vi "VNS IRH3T wOSSPClass.vi"(8 "error in (no error)":errorcluster, 10 "Best Chromosome In":u16[](array[numeric])=[1, 7, 8, 14, 6, 15, 11, 12, 3, 9, 5, 10, 4, 13, 0, 2], 11 "OSSP_Problem.lvclass":refnum<class "OSSP_Problem.lvclass">) -> (0 "error out":errorcluster, 1 "Tardiness(FIFO Engine)":u16, 2 "VNS Result":u16[](array[numeric]), 3 "OSSP_Problem out":refnum<class "OSSP_Problem.lvclass">)   [LabVIEW 2013]
uses:
  Classes/OSSP_Problem.lvclass
  Classes/OSSP_Problem.lvclass/OSSP_Problem.ctl
  GA/SubVIS/Remove Duplicates In Array.vi
  Classes/GanntChart_Class/Schedule and Create Gannt Chart.vi
  Classes/GanntChart_Class/Job Completion Times.vi
  Classes/GanntChart_Class/Reorder Chromosome  After Makespan Calculation.vi
  Classes/GanntChart_Class/Check Other Machines for Schedule Time.vi
  Classes/GanntChart_Class/Schedule Job.vi
  Classes/GanntChart_Class/Find Gaps on Particular Machine.vi
  Classes/GanntChart_Class/Increment Number of Jobs on Machine.vi
  Classes/GanntChart_Class/Operation to Machine Job Tuple.vi
  Classes/GanntChart_Class/Find Job On Other Machines.vi
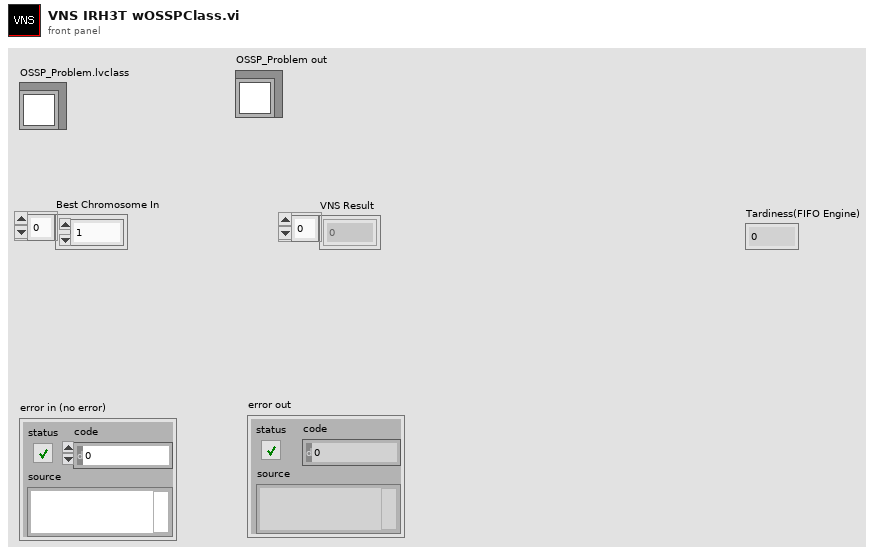
[diagram p1: front panel]
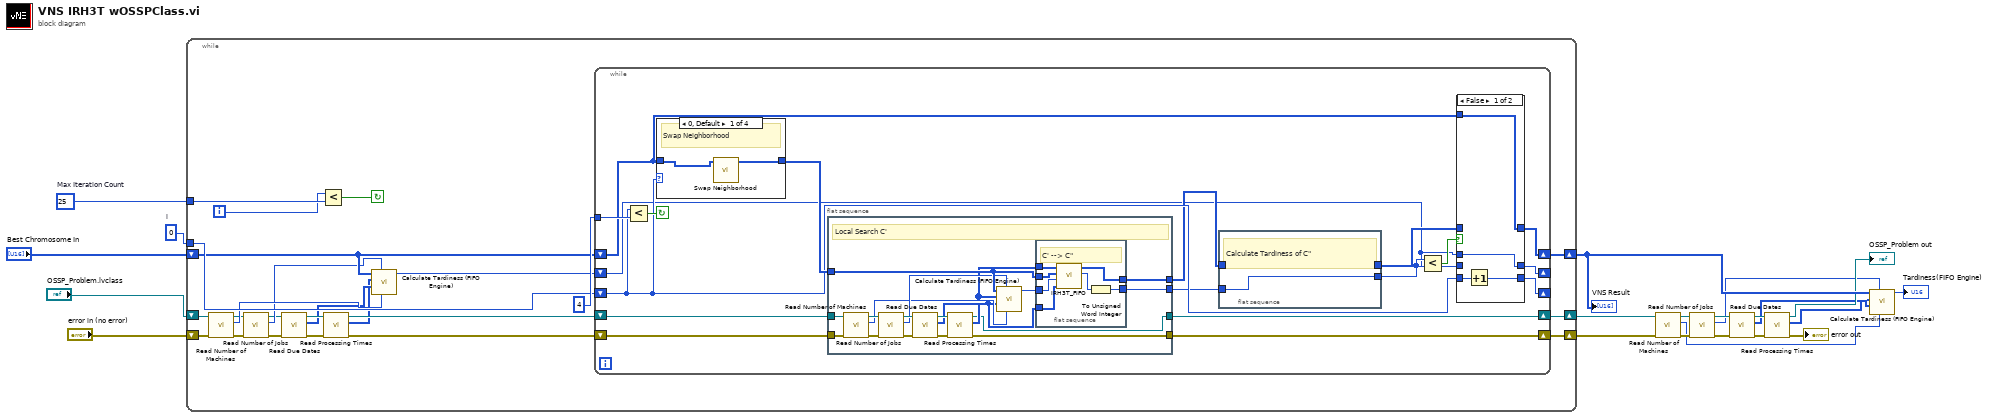
[diagram p0: block diagram]
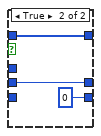
[diagram p2: hidden frame]
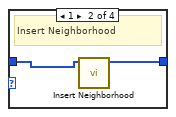
[diagram p3: hidden frame]
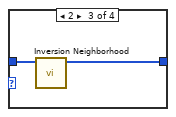
[diagram p4: hidden frame]
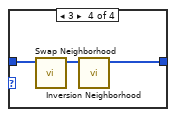
[diagram p5: hidden frame]
diagram:
  w20 = 0  # i
  w21 = 25  # Max Iteration Count
  n1 = while {
    tunnel: w21 -> [w45]
    tunnel: w20 -> [w42]
    shift-right: [w40] -> w19
    shift-left: "Best Chromosome In" -> [w33]
    shift-right: [w39] -> w10
    shift-left: "OSSP_Problem.lvclass" -> [w37]
    shift-right: [w38] -> w8
    shift-left: "error in (no error)" -> [w35]
    i -> [w41]
    stop <- w44 continue-if-true
    n2 = call-dynamic "Read Number of Machines.vi"("error in (no error)"=w35, "OSSP_Problem in"=w37) -> ("error out"=w30:errorcluster, "Number of Machines"=w32:i32, "OSSP_Problem out"=w31:refnum<class "OSSP_Problem.lvclass">)  [unwired: 7 in]
    n3 = call-dynamic "Read Number of Jobs.vi"("error in (no error)"=w30, "OSSP_Problem in"=w31) -> ("error out"=w27:errorcluster, "Number of Jobs"=w29:i32, "OSSP_Problem out"=w28:refnum<class "OSSP_Problem.lvclass">)  [unwired: 7 in]
    n4 = call "Read Due Dates.vi"("error in (no error)"=w27, "OSSP_Problem in"=w28) -> ("error out"=w26:errorcluster, "Due Dates"=w24:u16[], "OSSP_Problem out"=w25:refnum<class "OSSP_Problem.lvclass">)  [unwired: 7 in]
    n5 = Less?(x=w41, y=w45) -> (x < y?=w44:bool)
    n6 = call-dynamic "Read Processing Times.vi"("error in (no error)"=w26, "OSSP_Problem in"=w25) -> ("error out"=w34:errorcluster, "Processing Times"=w23:u16[][], "OSSP_Problem out"=w36:refnum<class "OSSP_Problem.lvclass">)  [unwired: 7 in]
    n7 = call "Calculate Tardiness (FIFO Engine).vi"("Number of Machines"=w32, "Number of Jobs"=w29, "Due Dates"=w24, "Processing Times"=w23, "Schedule In"=w33) -> ("Tardiness(FIFO Engine)"=w22:u16)  [unwired: 6 in]
    n8 = while {
      tunnel: 4 -> [w60]
      shift-right: [w59] -> _
      shift-left: w42 -> [w56]
      shift-right: [w58] -> w40
      shift-left: w33 -> [w57]
      shift-right: [w54] -> w39
      shift-left: w36 -> [w52]
      shift-right: [w53] -> w38
      shift-left: w34 -> [w51]
      shift-right: [w49] -> _
      shift-left: w22 -> [w46]
      stop <- w63 continue-if-true
      n9 = Less?(x=w56, y=w60) -> (x < y?=w63:bool)
      n10 = case shown="0, Default" w56 {
        tunnel: w57 -> [w99 w101 w103 w106]
        tunnel: [w98 w100 w102 w104] -> w62
        frame 0, Default {
          # "Swap Neighborhood"
          n11 = call "Swap Neighborhood.vi"("Schedule In"=w99) -> ("Schedule Out"=w98:u16[])  [unwired: 10 in]
        }
        frame 1 {
          # "Insert Neighborhood"
          n12 = call "Insert Neighborhood.vi"("C'"=w101) -> ("Best Chromosome In"=w100:u16[])  [unwired: 10 in]
        }
        frame 2 {
          n13 = call "Inversion Neighborhood.vi"("Schedule in"=w103) -> ("Schedule out"=w102:u16[])  [unwired: 10 in]
        }
        frame 3 {
          n14 = call "Swap Neighborhood.vi"("Schedule In"=w106) -> ("Schedule Out"=w105:u16[])  [unwired: 10 in]
          n15 = call "Inversion Neighborhood.vi"("Schedule in"=w105) -> ("Schedule out"=w104:u16[])  [unwired: 10 in]
        }
      }
      n16 = flat-sequence {
        tunnel: w62 -> [w89]
        tunnel: [w90] -> w48
        tunnel: [w87] -> w55
        tunnel: w52 -> [w80]
        tunnel: [w75] -> w54
        tunnel: w51 -> [w74]
        tunnel: [w73] -> w53
        frame #0 {
          # "Local Search C'"
          n17 = call-dynamic "Read Number of Machines.vi"("error in (no error)"=w74, "OSSP_Problem in"=w80) -> ("error out"=w85:errorcluster, "Number of Machines"=w78:i32, "OSSP_Problem out"=w86:refnum<class "OSSP_Problem.lvclass">)  [unwired: 7 in]
          n18 = call-dynamic "Read Number of Jobs.vi"("error in (no error)"=w85, "OSSP_Problem in"=w86) -> ("error out"=w83:errorcluster, "Number of Jobs"=w79:i32, "OSSP_Problem out"=w84:refnum<class "OSSP_Problem.lvclass">)  [unwired: 7 in]
          n19 = call "Read Due Dates.vi"("error in (no error)"=w83, "OSSP_Problem in"=w84) -> ("error out"=w82:errorcluster, "Due Dates"=w77:u16[], "OSSP_Problem out"=w81:refnum<class "OSSP_Problem.lvclass">)  [unwired: 7 in]
          n20 = call-dynamic "Read Processing Times.vi"("error in (no error)"=w82, "OSSP_Problem in"=w81) -> ("error out"=w73:errorcluster, "Processing Times"=w76:u16[][], "OSSP_Problem out"=w75:refnum<class "OSSP_Problem.lvclass">)  [unwired: 7 in]
          n21 = call "Calculate Tardiness (FIFO Engine).vi"("Number of Machines"=w78, "Number of Jobs"=w79, "Due Dates"=w77, "Processing Times"=w76, "Schedule In"=w89) -> ("Tardiness(FIFO Engine)"=w88:u16)  [unwired: 6 in]
          n22 = flat-sequence {
            tunnel: w89 -> [w97]
            tunnel: [w91] -> w90
            tunnel: w88 -> [w96]
            tunnel: w77 -> [w95]
            tunnel: [w92] -> w87
            tunnel: w76 -> [w94]
            frame #0 {
              # "C' --> C\""
              n23 = call "IRH3T_FIFO.vi"("Due Dates"=w95, "Initial Tardiness"=w96, "Schedule 2B Improved"=w97, "Proocessing Times  (Machines x Jobs)"=w94) -> ("Total Tardiness"=w93:i32, "IRH3T (Reordered) Schedule Out"=w91:u16[])  [unwired: 5 in, 1 out]
              n24 = To Unsigned Word Integer(number=w93) -> (unsigned 16bit integer=w92:u16)
            }
          }
        }
      }
      n25 = flat-sequence {
        tunnel: w48 -> [w64]
        tunnel: [w65] -> w50
        tunnel: w55 -> [w65]
        tunnel: [w64] -> w47
        frame #0 {
          # "Calculate Tardiness of C\""
        }
      }
      n26 = Less?(x=w50, y=w46) -> (x < y?=w61:bool)
      n27 = case shown="False" w61 {
        tunnel: w56 -> [w68 _]
        tunnel: w47 -> [_ w71]
        tunnel: [w69 0] -> w59
        tunnel: [w67 w71] -> w58
        tunnel: w57 -> [w67 _]
        tunnel: w50 -> [_ w70]
        tunnel: [w66 w70] -> w49
        tunnel: w46 -> [w66 _]
        frame False {
          n28 = Increment(x=w68) -> (x+1=w69:i32)
        }
        frame True {
        }
      }
    }
  }
  "VNS Result" <- w19
  n29 = call-dynamic "Read Number of Machines.vi"("error in (no error)"=w8, "OSSP_Problem in"=w10) -> ("error out"=w15:errorcluster, "Number of Machines"=w5:i32, "OSSP_Problem out"=w16:refnum<class "OSSP_Problem.lvclass">)  [unwired: 7 in]
  n30 = call-dynamic "Read Number of Jobs.vi"("error in (no error)"=w15, "OSSP_Problem in"=w16) -> ("error out"=w13:errorcluster, "Number of Jobs"=w4:i32, "OSSP_Problem out"=w14:refnum<class "OSSP_Problem.lvclass">)  [unwired: 7 in]
  n31 = call "Read Due Dates.vi"("error in (no error)"=w13, "OSSP_Problem in"=w14) -> ("error out"=w12:errorcluster, "Due Dates"=w3:u16[], "OSSP_Problem out"=w11:refnum<class "OSSP_Problem.lvclass">)  [unwired: 7 in]
  n32 = call-dynamic "Read Processing Times.vi"("error in (no error)"=w12, "OSSP_Problem in"=w11) -> ("error out"=→"error out":errorcluster, "Processing Times"=w2:u16[][], "OSSP_Problem out"=→"OSSP_Problem out":refnum<class "OSSP_Problem.lvclass">)  [unwired: 7 in]
  n33 = call "Calculate Tardiness (FIFO Engine).vi"("Number of Machines"=w5, "Number of Jobs"=w4, "Due Dates"=w3, "Processing Times"=w2, "Schedule In"=w19) -> ("Tardiness(FIFO Engine)"=→"Tardiness(FIFO Engine)":u16)  [unwired: 6 in]
